vi "Calculate Distances.vi"(8 "error in (no error)":errorcluster, 11 "Grassfire 2D In":refnum<class "Grassfire 2D.lvclass">) -> (0 "error out":errorcluster, 3 "Grassfire 2D Out":refnum<class "Grassfire 2D.lvclass">)   [LabVIEW 2019, in "Grassfire 2D.lvclass"]
uses:
  Grassfire 2D.lvclass
  Node Address--cluster.ctl
  Grassfire 2D.lvclass/Grassfire 2D.ctl
panel:
  out "Iteration Time":u32
  out "Total Time":u32
  out "i":i32
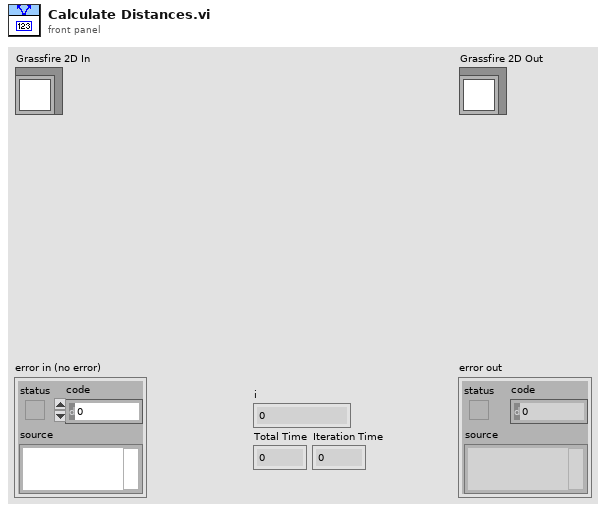
[diagram p1: front panel]
types:
  T1 = typedef "Grassfire 2D.lvclass/Node Address--cluster.ctl" = cluster{"Row":i32, "Column":i32}
  T2 = typedef "Grassfire 2D.lvclass/Node Value--cluster.ctl" = cluster{"Type":T3, "Distance":i32}
  T3 = typedef "Shared.lvlib/Node Type--enum.ctl" = enum16{"Empty", "Blocked", "Start", "End", "Path"}
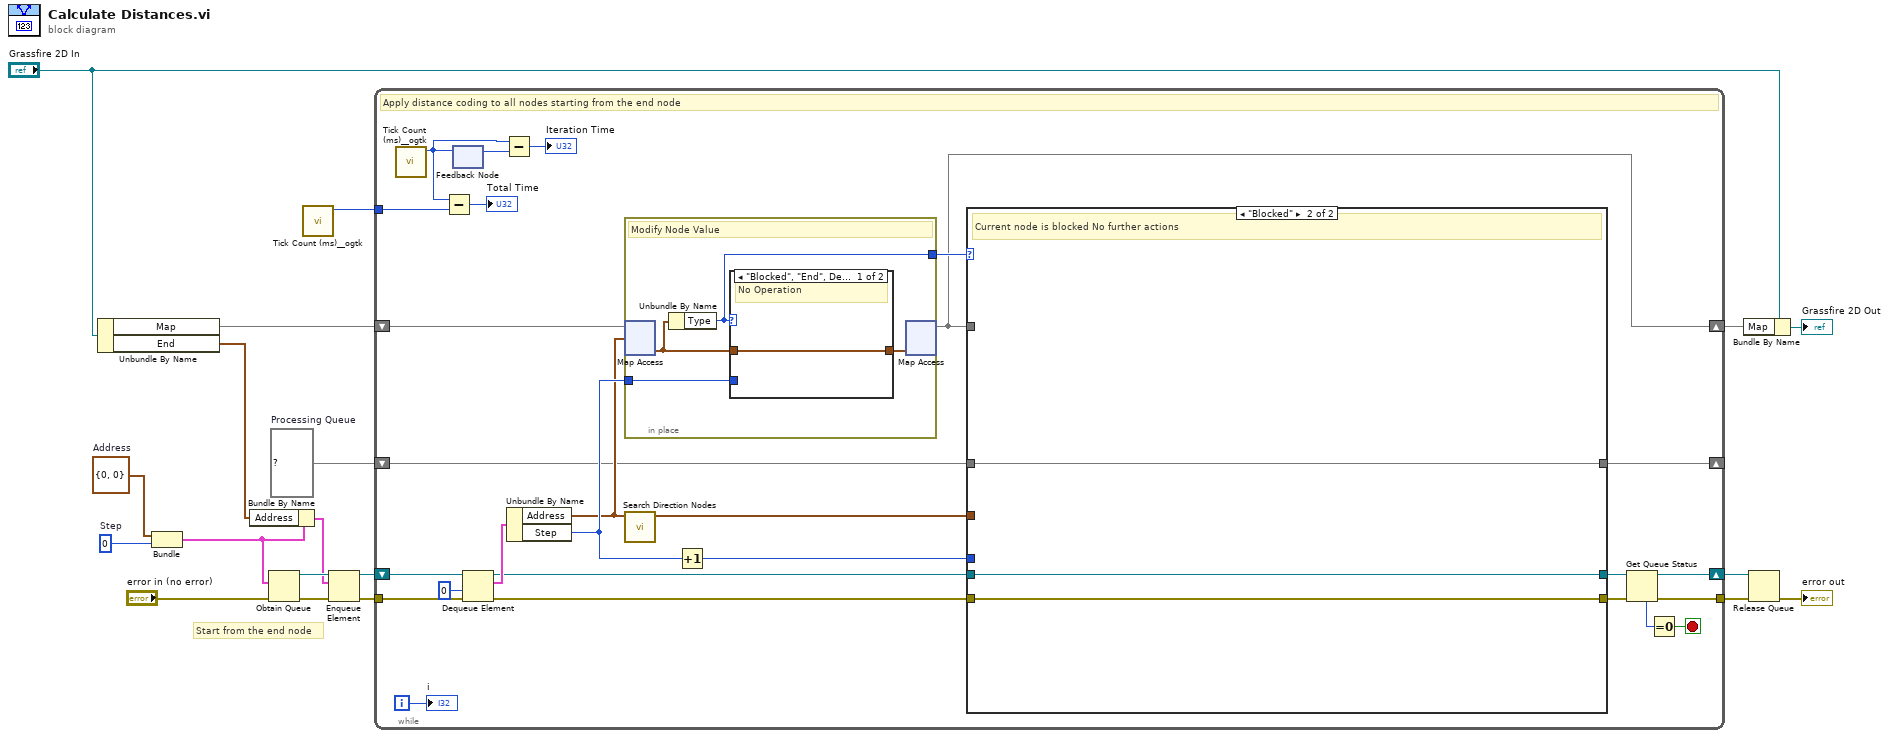
[diagram p0: block diagram]
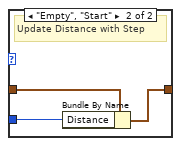
[diagram p2: hidden frame]
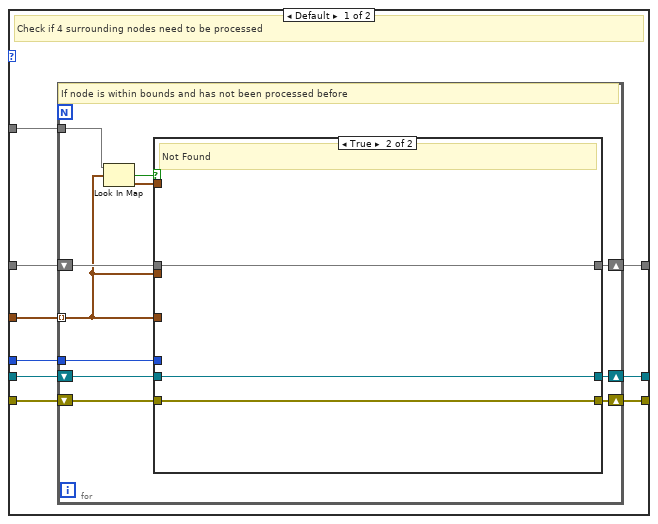
[diagram p3: hidden frame]
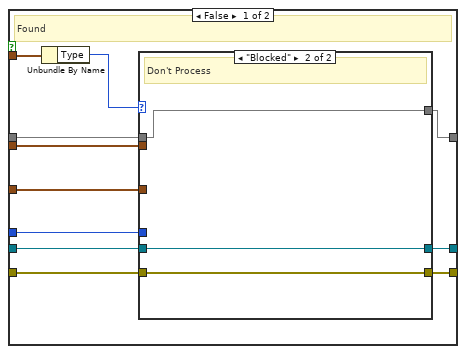
[diagram p4: hidden frame]
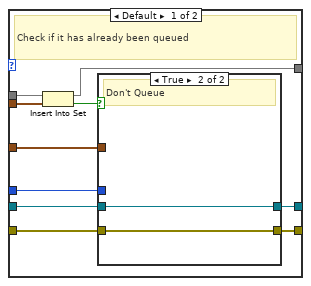
[diagram p5: hidden frame]
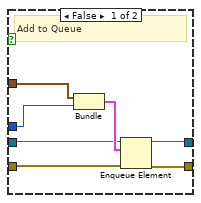
[diagram p6: hidden frame]
diagram:
  w2 = set{T1} {}  # Processing Queue
  w3 = T1 {"Row"=0, "Column"=0}  # Address
  w18 = 0  # Step
  # "Start from the end node"
  n1 = Unbundle By Name("Grassfire 2D In") -> ("Map"=w13:map{T1, T2}, "End"=w15:T1)
  n2 = Bundle("Address"=w3, "Step"=w18) -> (w17:cluster{"Address":T1, "Step":i32})  [unwired: 1 in]
  n3 = Bundle By Name(cluster=w17, "Address"=w15) -> (w16:cluster{"Address":T1, "Step":i32})
  n4 = Obtain Queue(element data type=w17, error in (no error)="error in (no error)") -> (queue out=w19:refnum<queue>, error out=w10:errorcluster)  [unwired: 3 in, 1 out]
  n5 = call <userlib>:"Tick Count (ms)__ogtk.vi"() -> ("millisecond timer value"=w1:u32)  [unwired: 10 in, 1 out]
  n6 = Enqueue Element(queue=w19, element=w16, error in (no error)=w10) -> (queue out=w11:refnum<queue>, error out=w12:errorcluster)  [unwired: 1 in, 1 out]
  n7 = while {
    shift-right: [w20] -> w7
    shift-left: w13 -> [w35]
    shift-right: [w39] -> w5
    shift-left: w11 -> [w45]
    tunnel: w12 -> [w42]
    tunnel: [w40] -> w6
    shift-right: [w22] -> _
    shift-left: w2 -> [w21]
    tunnel: w1 -> [w28]
    i -> [w29]
    stop <- w38 stop-if-true
    # "Apply distance coding to all nodes starting from the end node"
    n8 = call <userlib>:"Tick Count (ms)__ogtk.vi"() -> ("millisecond timer value"=w25:u32)  [unwired: 10 in, 1 out]
    n9 = Subtract(x=w25, y=w28) -> (x-y=→"Total Time":u32)
    n10 = feedback-in #1(w25) -> ()
    n11 = feedback #1() -> (w26:u32)  [unwired: 1 in]
    n12 = Dequeue Element(queue=w45, timeout in ms (-1)=0, error in (no error)=w42) -> (queue out=w43:refnum<queue>, element=w44:cluster{"Address":T1, "Step":i32}, error out=w41:errorcluster)  [unwired: 1 out]
    n13 = Subtract(x=w25, y=w26) -> (x-y=→"Iteration Time":u32)
    n14 = Unbundle By Name(w44) -> ("Address"=w31:T1, "Step"=w33:i32)
    n15 = in-place {
      in-place-border: w33 -> [w50]
      in-place-border: [w47] -> w34
      # "Modify Node Value"
      n16 = in-place-map #2(w35, w31) -> (w48:T2)  [unwired: 1 in, 1 out]
      n17 = Unbundle By Name(w48) -> ("Type"=w47:T3)
      n18 = case shown="\"Blocked\", \"End\", Default" w47 {
        tunnel: [w51 w53] -> w49
        tunnel: w48 -> [w51 w54]
        tunnel: w50 -> [_ w52]
        frame "Blocked", "End", Default {
          # "No Operation"
        }
        frame "Empty", "Start" {
          # "Update Distance with Step"
          n19 = Bundle By Name(cluster=w54, "Distance"=w52) -> (w53:T2)
        }
      }
      n20 = in-place-map #2(w49) -> (w20:map{T1, T2})  [unwired: 1 in, 2 out]
    }
    n21 = call "Search Direction Nodes.vi"("Address"=w31) -> ("Search Direction Nodes"=w30:T1[])  [unwired: 9 in, 1 out]
    n22 = Increment(x=w33) -> (x+1=w32:i32)
    n23 = case shown="\"Blocked\"" w34 {
      tunnel: [w62 w113] -> w37
      tunnel: w30 -> [w61 _]
      tunnel: w43 -> [w63 w113]
      tunnel: w41 -> [w60 w112]
      tunnel: [w59 w112] -> w36
      tunnel: w20 -> [w55 _]
      tunnel: w21 -> [w58 w111]
      tunnel: w32 -> [w57 _]
      tunnel: [w56 w111] -> w22
      frame Default {
        # "Check if 4 surrounding nodes need to be processed"
        n24 = for {
          tunnel: w61 -> [w70] mode=indexing
          shift-right: [w68] -> w62
          shift-left: w63 -> [w67]
          shift-right: [w66] -> w59
          shift-left: w60 -> [w65]
          tunnel: w57 -> [w69]
          shift-right: [w71] -> w56
          shift-left: w58 -> [w72]
          tunnel: w55 -> [w64]
          # "If node is within bounds and has not been processed before"
          n25 = Look In Map(map=w64, key=w70) -> (key not found?=w73:bool, value=w74:T2)  [unwired: 1 in]
          n26 = case shown="True" w73 {
            tunnel: w74 -> [w85 _]
            tunnel: w72 -> [w83 w110]
            tunnel: [w82 w110] -> w71
            tunnel: w70 -> [w81 _]
            tunnel: w70 -> [w80 _]
            tunnel: w69 -> [w79 _]
            tunnel: [w78 w109] -> w68
            tunnel: w67 -> [w77 w109]
            tunnel: [w76 w108] -> w66
            tunnel: w65 -> [w75 w108]
            frame False {
              # "Found"
              n27 = Unbundle By Name(w85) -> ("Type"=w84:T3)
              n28 = case shown="\"Blocked\"" w84 {
                tunnel: w83 -> [w95 w107]
                tunnel: [w93 w107] -> w82
                tunnel: w81 -> [w92 _]
                tunnel: w80 -> [w91 _]
                tunnel: w79 -> [w90 _]
                tunnel: [w89 w106] -> w78
                tunnel: w77 -> [w88 w106]
                tunnel: [w87 w105] -> w76
                tunnel: w75 -> [w86 w105]
                frame Default {
                  # "Check if it has already been queued"
                  n29 = Insert Into Set(10:w92, 11:w95) -> (2:w94:bool, 3:w93:set{T1})
                  n30 = case shown="True" w94 {
                    tunnel: w91 -> [w99 _]
                    tunnel: w90 -> [w98 _]
                    tunnel: [w101 w104] -> w89
                    tunnel: w88 -> [w97 w104]
                    tunnel: [w100 w103] -> w87
                    tunnel: w86 -> [w96 w103]
                    frame False {
                      # "Add to Queue"
                      n31 = Bundle("End"=w99, w98) -> (w102:cluster{"End":T1, i32})  [unwired: 1 in]
                      n32 = Enqueue Element(queue=w97, element=w102, error in (no error)=w96) -> (queue out=w101:refnum<queue>, error out=w100:errorcluster)  [unwired: 1 in, 1 out]
                    }
                    frame True {
                      # "Don't Queue"
                    }
                  }
                }
                frame "Blocked" {
                  # "Don't Process"
                }
              }
            }
            frame True {
              # "Not Found"
            }
          }
        }
      }
      frame "Blocked" {
        # "Current node is blocked No further actions"
      }
    }
    n33 = Get Queue Status(queue=w37, error in (no error)=w36) -> (queue out=w39:refnum<queue>, error out=w40:errorcluster, # elements in queue=w23:i32)  [unwired: 1 in, 5 out]
    n34 = Equal To 0?(x=w23) -> (x = 0?=w38:bool)
    "i" <- w29
  }
  n35 = Bundle By Name(cluster="Grassfire 2D In", "Map"=w7) -> (→"Grassfire 2D Out":refnum<class "Grassfire 2D.lvclass">)
  n36 = Release Queue(queue=w5, error in (no error)=w6) -> (error out=→"error out":errorcluster)  [unwired: 1 in, 2 out]
